vi "Create_Trajectory_Config_Parse_V1_V2_V3.vi"(8 "error in (no error)":errorcluster, 10 "Units Selector":T4, 11 "XML Elements":string) -> (0 "error out":errorcluster, 3 "TrajCreateConfig":T1 {"WayPoints"."WEIGHT" format="%13.3f"; "WayPoints"."ANGLE" format="%13.3f"; "WayPoints"."Y" format="%13.3f"; "WayPoints"."X" format="%13.3f"; "TRAJECTORY_CONFIG"."End Velocity" format="%20.4f"; "TRAJECTORY_CONFIG"."StartVelocity" format="%20.4f"; "TRAJECTORY_CONFIG"."Max Acceleration" format="%20.4f"; "TRAJECTORY_CONFIG"."MaxVelocity" format="%20.4f"})   [LabVIEW 2019]
uses:
  TrajCreateUnitsENUM.ctl
  TrajCreateConfig__V_Internal.ctl
  <vilib>/Rock Robotics/WPI/ThirdParty/JAS_Junk/TrajLib/DISPLAY_WEIGHTED_WAYPOINT.ctl
  <vilib>/Rock Robotics/WPI/ThirdParty/JAS_Junk/TrajLib/TRAJ_CONFIG.ctl
  TrajCreateConfig_V4.ctl
  TrajCreateTrajConfig_V4.ctl
  <vilib>/Rock Robotics/WPI/ThirdParty/JAS_Junk/TrajLib/TRAJ_CONSTRAINT_DIIF_DRIVE_KINEMATICS.ctl
  <vilib>/Rock Robotics/WPI/ThirdParty/JAS_Junk/TrajLib/DIFF_DRIVE_KINEMATICS.ctl
  <vilib>/Rock Robotics/WPI/ThirdParty/JAS_Junk/TrajLib/TRAJ_CONSTRAINT_CENTRIPETAL_ACCEL.ctl
  <vilib>/Rock Robotics/WPI/ThirdParty/JAS_Junk/TrajLib/TRAJ_CONSTRAINT_SWERVE_DRIVE_KINEMATICS.ctl
  <vilib>/Rock Robotics/WPI/ThirdParty/JAS_Junk/TrajLib/SWERVE_DRIVE_KINEMATICS.ctl
  <vilib>/Analysis/Matrix/Datatypes/RealMatrix.ctl
  <vilib>/Rock Robotics/WPI/ThirdParty/JAS_Junk/TrajLib/TRANSLATION2D.ctl
  <vilib>/Rock Robotics/WPI/ThirdParty/JAS_Junk/TrajLib/TRAJ_CONSTRAINT_DIIF_DRIVE_VOLTAGE.ctl
  <vilib>/Rock Robotics/WPI/ThirdParty/JAS_Junk/TrajLib/SIMPLE_MOTOR_FF.ctl
  <vilib>/Rock Robotics/WPI/ThirdParty/JAS_Junk/TrajLib/TRAJ_CONSTRAINT_MECA_DRIVE_KINEMATICS.ctl
  <vilib>/Rock Robotics/WPI/ThirdParty/JAS_Junk/TrajLib/MECA_DRIVE_KINEMATICS.ctl
  TrajCreateConfig_V3.ctl
  TrajCreateConfig_V2.ctl
  <vilib>/Rock Robotics/WPI/ThirdParty/JAS_Junk/TrajLib/DISPLAY_WAYPOINT.ctl
  TrajCreateConfig_V1.ctl
  <vilib>/Rock Robotics/WPI/ThirdParty/JAS_Junk/TrajLib/Trajectory_Library.lvlib
  <vilib>/Analysis/Matrix/NI_Matrix.lvlib
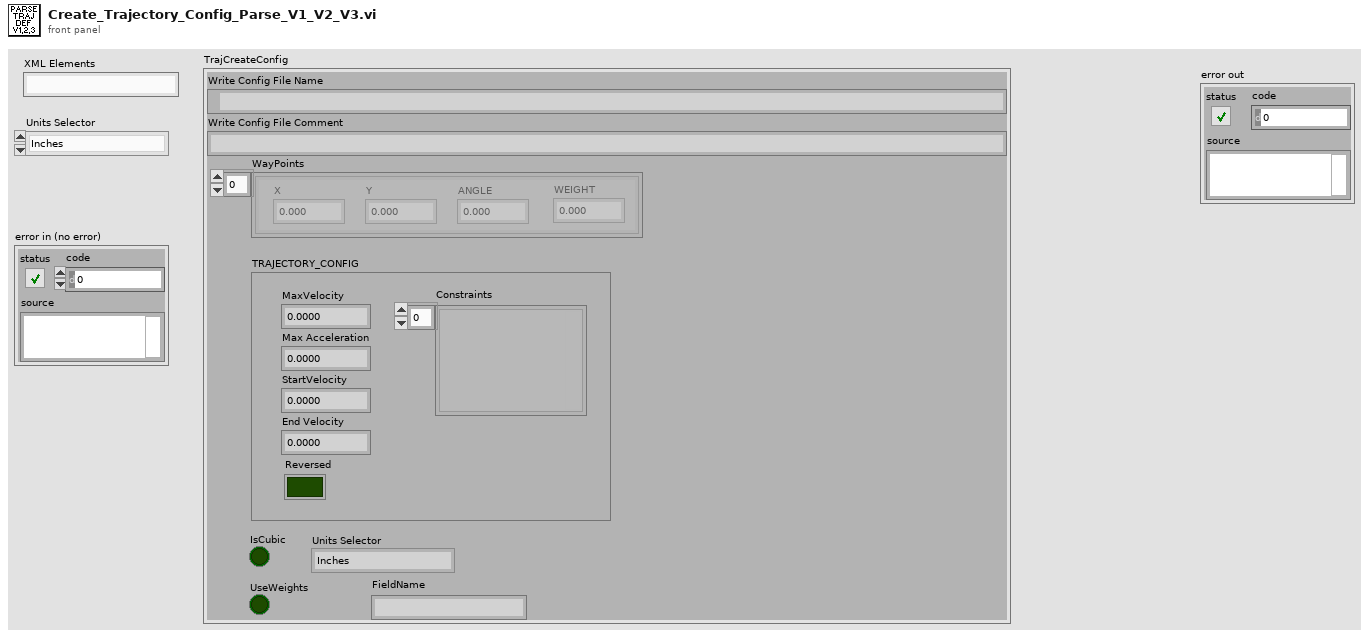
[diagram p1: front panel]
types:
  T1 = typedef "TrajCreateConfig__V_Internal.ctl" = cluster{"Write Config File Name":path, "Write Config File Comment":string, "WayPoints":T2[], "TRAJECTORY_CONFIG":T3, "IsCubic":bool, "Units Selector":T4, "UseWeights":bool, "FieldName":string}
  T2 = typedef "Trajectory_Library.lvlib/DISPLAY_WEIGHTED_WAYPOINT.ctl" = cluster{"X":dbl, "Y":dbl, "ANGLE":dbl, "WEIGHT":dbl}
  T3 = typedef "Trajectory_Library.lvlib/TRAJ_CONFIG.ctl" = cluster{"MaxVelocity":dbl, "Max Acceleration":dbl, "StartVelocity":dbl, "End Velocity":dbl, "Reversed":bool, "Constraints":variant[]}
  T4 = typedef "TrajCreateUnitsENUM.ctl" = enum16{"Inches", "Feet", "Centimeters", "Meters"}
  T5 = typedef "TrajCreateConfig_V4.ctl" = cluster{"Write Config File Name":path, "Write Config File Comment":string, "WayPoints":T2[], "TRAJECTORY_CONFIG_V4":T6, "IsCubic":bool, "Units Selector":T4, "UseWeights":bool, "FieldName":string}
  T6 = typedef "TrajCreateTrajConfig_V4.ctl" = cluster{"MaxVelocity":dbl, "Max Acceleration":dbl, "StartVelocity":dbl, "End Velocity":dbl, "Reversed":bool, "DiffDrKineConstntDefined":bool, "CentAcellConstntDefined":bool, "DiffDrVoltConstntDefined":bool, "DIFF_DRIVE_KINE_CONSTRAINT":T7, "CENTRIPETAL_ACCEL_CONSTRAINT":T9, "SwerveDrKineConstntDefined":bool, "SWERVE_DRIVE_KINE_CONSTRAINT":T10, "DIFF_DRIVE_VOLTAGE_CONSTRAINT":T14, "MECANUM_DRIVE_KINE_CONSTRAINT":T16, "MecanumDrKineConstntDefined":bool}
  T7 = typedef "Trajectory_Library.lvlib/TRAJ_CONSTRAINT_DIIF_DRIVE_KINEMATICS.ctl" = cluster{"Max Speed (M/S)":dbl, "DIFF_DRIVE_KINEMATICS":T8, "Max Accel (M/S2)":dbl}
  T8 = typedef "Trajectory_Library.lvlib/DIFF_DRIVE_KINEMATICS.ctl" = cluster{"TrackWidth_Meters":dbl}
  T9 = typedef "Trajectory_Library.lvlib/TRAJ_CONSTRAINT_CENTRIPETAL_ACCEL.ctl" = cluster{"Max Cent Accel":dbl}
  T10 = typedef "Trajectory_Library.lvlib/TRAJ_CONSTRAINT_SWERVE_DRIVE_KINEMATICS.ctl" = cluster{"Max Speed (M/S)":dbl, "SwerveKinematics":T11}
  T11 = typedef "Trajectory_Library.lvlib/SWERVE_DRIVE_KINEMATICS.ctl" = cluster{"NumModules":i32, "InverseKinematics":T12, "ForwardKinematics":T12, "Modules":T13[], "PrevCoR":T13}
  T12 = typedef "NI_Matrix.lvlib/RealMatrix.ctl" = dbl[][]
  T13 = typedef "Trajectory_Library.lvlib/TRANSLATION2D.ctl" = cluster{"X":dbl, "Y":dbl}
  T14 = typedef "Trajectory_Library.lvlib/TRAJ_CONSTRAINT_DIIF_DRIVE_VOLTAGE.ctl" = cluster{"Max Voltage":dbl, "DIFF_DRIVE_KINEMATICS":T8, "SIMPLE_MOTOR_FF":T15}
  T15 = typedef "Trajectory_Library.lvlib/SIMPLE_MOTOR_FF.ctl" = cluster{"Ks":dbl, "Kv":dbl, "Ka":dbl}
  T16 = typedef "Trajectory_Library.lvlib/TRAJ_CONSTRAINT_MECA_DRIVE_KINEMATICS.ctl" = cluster{"Max Speed (M/S)":dbl, "MECA_DRIVE_KINEMATICS":T17}
  T17 = typedef "Trajectory_Library.lvlib/MECA_DRIVE_KINEMATICS.ctl" = cluster{"FrontLeft":T13, "FrontRight":T13, "RearLeft":T13, "RearRight":T13, "InverseKinematics":T12, "ForwardKinematics":T12, "PrevCoR":T13}
  T18 = typedef "TrajCreateConfig_V3.ctl" = cluster{"Write Config File Name":path, "Write Config File Comment":string, "WayPoints":T2[], "TRAJECTORY_CONFIG":cluster{"MaxVelocity":dbl, "Max Acceleration":dbl, "StartVelocity":dbl, "End Velocity":dbl, "Reversed":bool, "DiffDrKineConstntDefined":bool, "CentAcellConstntDefined":bool, "DiffDrVoltConstntDefined":bool, "DIFF_DRIVE_KINE_CONSTRAINT":cluster{"Max Speed (M/S)":dbl, "DIFF_DRIVE_KINEMATICS":T8}, "CENTRIPETAL_ACCEL_CONSTRAINT":T9, "SwerveDrKineConstntDefined":bool, "SWERVE_DRIVE_KINE_CONSTRAINT":T10, "DIFF_DRIVE_VOLTAGE_CONSTRAINT":T14, "MECANUM_DRIVE_KINE_CONSTRAINT":T16, "MecanumDrKineConstntDefined":bool}, "IsCubic":bool, "Units Selector":T4, "UseWeights":bool}
  T19 = typedef "TrajCreateConfig_V2.ctl" = cluster{"Write Config File Name":path, "Write Config File Comment":string, "WayPoints":T20[], "TRAJECTORY_CONFIG":cluster{"MaxVelocity":dbl, "Max Acceleration":dbl, "StartVelocity":dbl, "End Velocity":dbl, "Reversed":bool, "DiffDrKineConstntDefined":bool, "CentAcellConstntDefined":bool, "DiffDrVoltConstntDefined":bool, "DIFF_DRIVE_KINE_CONSTRAINT":cluster{"Max Speed (M/S)":dbl, "DIFF_DRIVE_KINEMATICS":T8}, "CENTRIPETAL_ACCEL_CONSTRAINT":T9, "SwerveDrKineConstntDefined":bool, "SWERVE_DRIVE_KINE_CONSTRAINT":T10, "DIFF_DRIVE_VOLTAGE_CONSTRAINT":T14, "MECANUM_DRIVE_KINE_CONSTRAINT":T16, "MecanumDrKineConstntDefined":bool}, "IsCubic":bool, "Units Selector":T4}
  T20 = typedef "Trajectory_Library.lvlib/DISPLAY_WAYPOINT.ctl" = cluster{"X":dbl, "Y":dbl, "ANGLE":dbl}
  T21 = typedef "TrajCreateConfig_V1.ctl" = cluster{"Write Config File Name":path, "Write Config File Comment":string, "WayPoints":T20[], "TRAJECTORY_CONFIG":cluster{"MaxVelocity":dbl, "Max Acceleration":dbl, "StartVelocity":dbl, "End Velocity":dbl, "Reversed":bool, "DiffDrKineConstntDefined":bool, "CentAcellConstntDefined":bool, "DiffDrVoltConstntDefined":bool, "DIFF_DRIVE_KINE_CONSTRAINT":cluster{"Max Speed (M/S)":dbl, "DIFF_DRIVE_KINEMATICS":T8}, "CENTRIPETAL_ACCEL_CONSTRAINT":T9, "SwerveDrKineConstntDefined":bool, "SWERVE_DRIVE_KINE_CONSTRAINT":T10, "DIFF_DRIVE_VOLTAGE_CONSTRAINT":T14, "MECANUM_DRIVE_KINE_CONSTRAINT":T16, "MecanumDrKineConstntDefined":bool}, "IsCubic":bool}
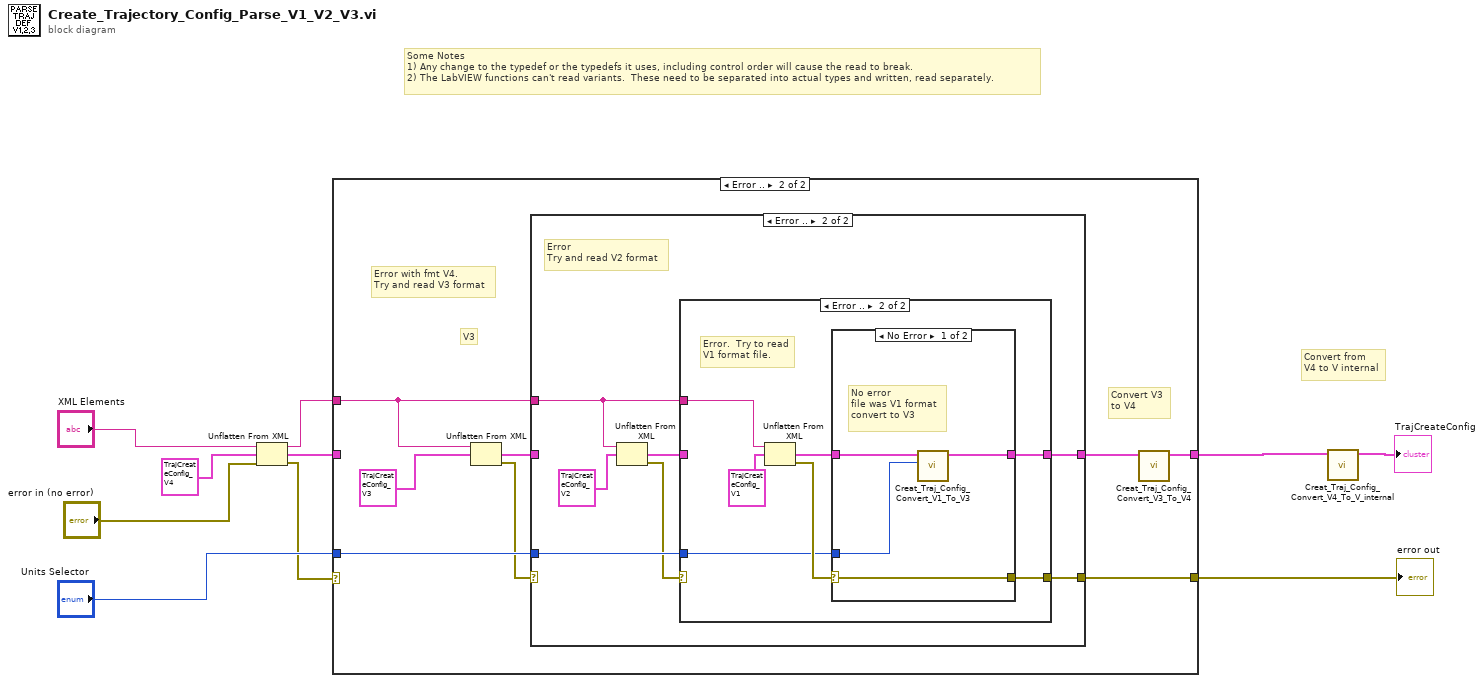
[diagram p0: block diagram]
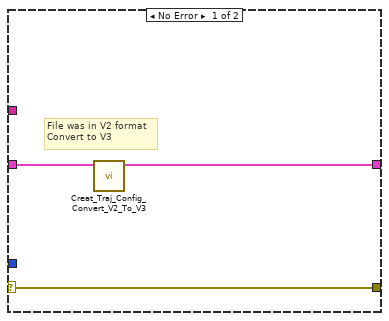
[diagram p4: hidden frame]
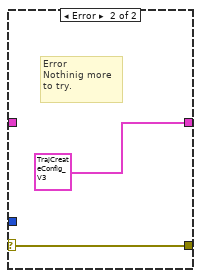
[diagram p5: hidden frame]
diagram:
  # "Convert from\nV4 to V internal"
  # "Some Notes\n1) Any change to the typedef or the typedefs it uses, including control order will cause the read to break.\n2) The LabVIEW functions can't read variants.  These need to be separated into actual types and written, read separately."
  n1 = Unflatten From XML(xml string="XML Elements", type=T5 {"Write Config File Name"=path "", "Write Config File Comment"="", "WayPoints"=[], "TRAJECTORY_CONFIG_V4"={"MaxVelocity"=0.0, "Max Acceleration"=0.0, "StartVelocity"=0.0, "End Velocity"=0.0, "Reversed"=FALSE, "DiffDrKineConstntDefined"=FALSE, "CentAcellConstntDefined"=FALSE, "DiffDrVoltConstntDefined"=FALSE, "DIFF_DRIVE_KINE_CONSTRAINT"={"Max Speed (M/S)"=0.0, "DIFF_DRIVE_KINEMATICS"={"TrackWidth_Meters"=0.0}, "Max Accel (M/S2)"=99999.0}, "CENTRIPETAL_ACCEL_CONSTRAINT"={"Max Cent Accel"=0.0}, "SwerveDrKineConstntDefined"=FALSE, "SWERVE_DRIVE_KINE_CONSTRAINT"={"Max Speed (M/S)"=0.0, "SwerveKinematics"={"NumModules"=0, "InverseKinematics"=[], "ForwardKinematics"=[], "Modules"=[], "PrevCoR"={"X"=0.0, "Y"=0.0}}}, "DIFF_DRIVE_VOLTAGE_CONSTRAINT"={"Max Voltage"=0.0, "DIFF_DRIVE_KINEMATICS"={"TrackWidth_Meters"=0.0}, "SIMPLE_MOTOR_FF"={"Ks"=0.0, "Kv"=0.0, "Ka"=0.0}}, "MECANUM_DRIVE_KINE_CONSTRAINT"={"Max Speed (M/S)"=0.0, "MECA_DRIVE_KINEMATICS"={"FrontLeft"={"X"=0.0, "Y"=0.0}, "FrontRight"={"X"=0.0, "Y"=0.0}, "RearLeft"={"X"=0.0, "Y"=0.0}, "RearRight"={"X"=0.0, "Y"=0.0}, "InverseKinematics"=[[0.0, 1.0, -1.0, 0.0], [0.0, 1.0, 1.0, 0.0], [0.0, 1.0, 1.0, 0.0], [0.0, 1.0, -1.0, 0.0]], "ForwardKinematics"=[[0.0, 1.0, -1.0, 0.0], [0.0, 1.0, 1.0, 0.0], [0.0, 1.0, 1.0, 0.0], [0.0, 1.0, -1.0, 0.0]], "PrevCoR"={"X"=0.0, "Y"=0.0}}}, "MecanumDrKineConstntDefined"=FALSE}, "IsCubic"=FALSE, "Units Selector"=enum."Inches", "UseWeights"=FALSE, "FieldName"=""} ("TrajCreateConfig"), error in (no error)="error in (no error)") -> (value=w3:T5, error out=w5:errorcluster)
  n2 = case shown="Error .." w5 {
    selector: w5 -> [w10 _]
    tunnel: "Units Selector" -> [_ w19]
    tunnel: [w10 w18] -> w8
    tunnel: "XML Elements" -> [_ w14]
    tunnel: [w11 w12] -> w1
    tunnel: w3 -> [w11 _]
    frame No Error {
      # "No Error -- File was in V4 Format"
    }
    frame Error {
      # "Convert V3\nto V4"
      # "Error with fmt V4.\nTry and read V3 format"
      # "V3"
      n3 = Unflatten From XML(xml string=w14, type=T18 {"Write Config File Name"=path "", "Write Config File Comment"="", "WayPoints"=[], "TRAJECTORY_CONFIG"={"MaxVelocity"=0.0, "Max Acceleration"=0.0, "StartVelocity"=0.0, "End Velocity"=0.0, "Reversed"=FALSE, "DiffDrKineConstntDefined"=FALSE, "CentAcellConstntDefined"=FALSE, "DiffDrVoltConstntDefined"=FALSE, "DIFF_DRIVE_KINE_CONSTRAINT"={"Max Speed (M/S)"=0.0, "DIFF_DRIVE_KINEMATICS"={"TrackWidth_Meters"=0.0}}, "CENTRIPETAL_ACCEL_CONSTRAINT"={"Max Cent Accel"=0.0}, "SwerveDrKineConstntDefined"=FALSE, "SWERVE_DRIVE_KINE_CONSTRAINT"={"Max Speed (M/S)"=0.0, "SwerveKinematics"={"NumModules"=0, "InverseKinematics"=[], "ForwardKinematics"=[], "Modules"=[], "PrevCoR"={"X"=0.0, "Y"=0.0}}}, "DIFF_DRIVE_VOLTAGE_CONSTRAINT"={"Max Voltage"=0.0, "DIFF_DRIVE_KINEMATICS"={"TrackWidth_Meters"=0.0}, "SIMPLE_MOTOR_FF"={"Ks"=0.0, "Kv"=0.0, "Ka"=0.0}}, "MECANUM_DRIVE_KINE_CONSTRAINT"={"Max Speed (M/S)"=0.0, "MECA_DRIVE_KINEMATICS"={"FrontLeft"={"X"=0.0, "Y"=0.0}, "FrontRight"={"X"=0.0, "Y"=0.0}, "RearLeft"={"X"=0.0, "Y"=0.0}, "RearRight"={"X"=0.0, "Y"=0.0}, "InverseKinematics"=[], "ForwardKinematics"=[], "PrevCoR"={"X"=0.0, "Y"=0.0}}}, "MecanumDrKineConstntDefined"=FALSE}, "IsCubic"=FALSE, "Units Selector"=enum."Inches", "UseWeights"=FALSE} ("TrajCreateConfig")) -> (value=w16:T18, error out=w15:errorcluster)  [unwired: 1 in]
      n4 = case shown="Error .." w15 {
        selector: w15 -> [w21 _]
        tunnel: [w21 w24] -> w18
        tunnel: w19 -> [_ w26]
        tunnel: w16 -> [w20 _]
        tunnel: [w20 w23] -> w13
        tunnel: w14 -> [_ w22]
        frame No Error {
          # "No Error.  File was V3\nformat."
        }
        frame Error {
          # "Error\nTry and read V2 format"
          n5 = Unflatten From XML(xml string=w22, type=T19 {"Write Config File Name"=path "", "Write Config File Comment"="", "WayPoints"=[], "TRAJECTORY_CONFIG"={"MaxVelocity"=0.0, "Max Acceleration"=0.0, "StartVelocity"=0.0, "End Velocity"=0.0, "Reversed"=FALSE, "DiffDrKineConstntDefined"=FALSE, "CentAcellConstntDefined"=FALSE, "DiffDrVoltConstntDefined"=FALSE, "DIFF_DRIVE_KINE_CONSTRAINT"={"Max Speed (M/S)"=0.0, "DIFF_DRIVE_KINEMATICS"={"TrackWidth_Meters"=0.0}}, "CENTRIPETAL_ACCEL_CONSTRAINT"={"Max Cent Accel"=0.0}, "SwerveDrKineConstntDefined"=FALSE, "SWERVE_DRIVE_KINE_CONSTRAINT"={"Max Speed (M/S)"=0.0, "SwerveKinematics"={"NumModules"=0, "InverseKinematics"=[], "ForwardKinematics"=[], "Modules"=[], "PrevCoR"={"X"=0.0, "Y"=0.0}}}, "DIFF_DRIVE_VOLTAGE_CONSTRAINT"={"Max Voltage"=0.0, "DIFF_DRIVE_KINEMATICS"={"TrackWidth_Meters"=0.0}, "SIMPLE_MOTOR_FF"={"Ks"=0.0, "Kv"=0.0, "Ka"=0.0}}, "MECANUM_DRIVE_KINE_CONSTRAINT"={"Max Speed (M/S)"=0.0, "MECA_DRIVE_KINEMATICS"={"FrontLeft"={"X"=0.0, "Y"=0.0}, "FrontRight"={"X"=0.0, "Y"=0.0}, "RearLeft"={"X"=0.0, "Y"=0.0}, "RearRight"={"X"=0.0, "Y"=0.0}, "InverseKinematics"=[], "ForwardKinematics"=[], "PrevCoR"={"X"=0.0, "Y"=0.0}}}, "MecanumDrKineConstntDefined"=FALSE}, "IsCubic"=FALSE, "Units Selector"=enum."Inches"} ("TrajCreateConfig")) -> (value=w27:T19, error out=w25:errorcluster)  [unwired: 1 in]
          n6 = case shown="Error .." w25 {
            selector: w25 -> [w30 _]
            tunnel: w27 -> [w31 _]
            tunnel: w26 -> [_ w33]
            tunnel: [w30 w35] -> w24
            tunnel: [w29 w34] -> w23
            tunnel: w22 -> [_ w37]
            frame No Error {
              # "File was in V2 format\nConvert to V3"
              n7 = call "Creat_Traj_Config_Convert_V2_To_V3.vi"("TrajCreateConfig in"=w31) -> ("TrajCreateConfig out"=w29:T18)  [unwired: 10 in]
            }
            frame Error {
              # "Error.  Try to read\nV1 format file."
              n8 = Unflatten From XML(xml string=w37, type=T21 {"Write Config File Name"=path "", "Write Config File Comment"="", "WayPoints"=[], "TRAJECTORY_CONFIG"={"MaxVelocity"=0.0, "Max Acceleration"=0.0, "StartVelocity"=0.0, "End Velocity"=0.0, "Reversed"=FALSE, "DiffDrKineConstntDefined"=FALSE, "CentAcellConstntDefined"=FALSE, "DiffDrVoltConstntDefined"=FALSE, "DIFF_DRIVE_KINE_CONSTRAINT"={"Max Speed (M/S)"=0.0, "DIFF_DRIVE_KINEMATICS"={"TrackWidth_Meters"=0.0}}, "CENTRIPETAL_ACCEL_CONSTRAINT"={"Max Cent Accel"=0.0}, "SwerveDrKineConstntDefined"=FALSE, "SWERVE_DRIVE_KINE_CONSTRAINT"={"Max Speed (M/S)"=0.0, "SwerveKinematics"={"NumModules"=0, "InverseKinematics"=[], "ForwardKinematics"=[], "Modules"=[], "PrevCoR"={"X"=0.0, "Y"=0.0}}}, "DIFF_DRIVE_VOLTAGE_CONSTRAINT"={"Max Voltage"=0.0, "DIFF_DRIVE_KINEMATICS"={"TrackWidth_Meters"=0.0}, "SIMPLE_MOTOR_FF"={"Ks"=0.0, "Kv"=0.0, "Ka"=0.0}}, "MECANUM_DRIVE_KINE_CONSTRAINT"={"Max Speed (M/S)"=0.0, "MECA_DRIVE_KINEMATICS"={"FrontLeft"={"X"=0.0, "Y"=0.0}, "FrontRight"={"X"=0.0, "Y"=0.0}, "RearLeft"={"X"=0.0, "Y"=0.0}, "RearRight"={"X"=0.0, "Y"=0.0}, "InverseKinematics"=[], "ForwardKinematics"=[], "PrevCoR"={"X"=0.0, "Y"=0.0}}}, "MecanumDrKineConstntDefined"=FALSE}, "IsCubic"=FALSE} ("TrajCreateConfig")) -> (value=w32:T21, error out=w36:errorcluster)  [unwired: 1 in]
              n9 = case shown="No Error" w36 {
                selector: w36 -> [w42 w44]
                tunnel: [w42 w44] -> w35
                tunnel: [w41 T18 {"Write Config File Name"=path "", "Write Config File Comment"="", "WayPoints"=[], "TRAJECTORY_CONFIG"={"MaxVelocity"=0.0, "Max Acceleration"=0.0, "StartVelocity"=0.0, "End Velocity"=0.0, "Reversed"=FALSE, "DiffDrKineConstntDefined"=FALSE, "CentAcellConstntDefined"=FALSE, "DiffDrVoltConstntDefined"=FALSE, "DIFF_DRIVE_KINE_CONSTRAINT"={"Max Speed (M/S)"=0.0, "DIFF_DRIVE_KINEMATICS"={"TrackWidth_Meters"=0.0}}, "CENTRIPETAL_ACCEL_CONSTRAINT"={"Max Cent Accel"=0.0}, "SwerveDrKineConstntDefined"=FALSE, "SWERVE_DRIVE_KINE_CONSTRAINT"={"Max Speed (M/S)"=0.0, "SwerveKinematics"={"NumModules"=0, "InverseKinematics"=[], "ForwardKinematics"=[], "Modules"=[], "PrevCoR"={"X"=0.0, "Y"=0.0}}}, "DIFF_DRIVE_VOLTAGE_CONSTRAINT"={"Max Voltage"=0.0, "DIFF_DRIVE_KINEMATICS"={"TrackWidth_Meters"=0.0}, "SIMPLE_MOTOR_FF"={"Ks"=0.0, "Kv"=0.0, "Ka"=0.0}}, "MECANUM_DRIVE_KINE_CONSTRAINT"={"Max Speed (M/S)"=0.0, "MECA_DRIVE_KINEMATICS"={"FrontLeft"={"X"=0.0, "Y"=0.0}, "FrontRight"={"X"=0.0, "Y"=0.0}, "RearLeft"={"X"=0.0, "Y"=0.0}, "RearRight"={"X"=0.0, "Y"=0.0}, "InverseKinematics"=[], "ForwardKinematics"=[], "PrevCoR"={"X"=0.0, "Y"=0.0}}}, "MecanumDrKineConstntDefined"=FALSE}, "IsCubic"=FALSE, "Units Selector"=enum."Inches", "UseWeights"=FALSE} ("TrajCreateConfig")] -> w34
                tunnel: w33 -> [w40 _]
                tunnel: w32 -> [w39 _]
                frame No Error {
                  # "No error\nfile was V1 format\nconvert to V3"
                  n10 = call "Creat_Traj_Config_Convert_V1_To_V3.vi"("Units Selector"=w40, "TrajCreateConfig in"=w39) -> ("TrajCreateConfig out"=w41:T18)  [unwired: 9 in]
                }
                frame Error {
                  # "Error\nNothinig more\nto try."
                }
              }
            }
          }
        }
      }
      n11 = call "Creat_Traj_Config_Convert_V3_To_V4.vi"("TrajCreateConfig in"=w13) -> ("TrajCreateConfig out"=w12:T5)  [unwired: 10 in]
    }
  }
  "error out" <- w8
  n12 = call "Creat_Traj_Config_Convert_V4_To_V_internal.vi"("TrajCreateConfig V4"=w1) -> ("TrajCreateConfig V_Internal"=→"TrajCreateConfig":T1)  [unwired: 10 in]
